vi "EnumeratorUnderstanding.vi"() -> ()   [LabVIEW 2019]
panel:
  out "Value of Enum":enum16{"First ", "Second", "third", ""}(ring)
  in  "Enum":enum16{"First ", "Second", "third", ""}(ring)
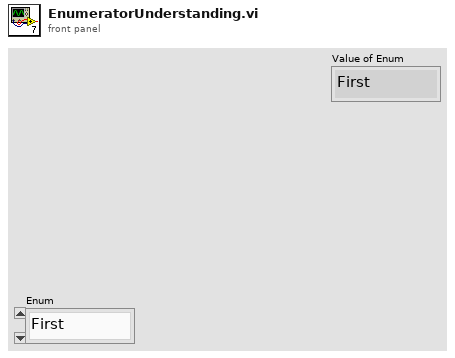
[diagram p1: front panel]
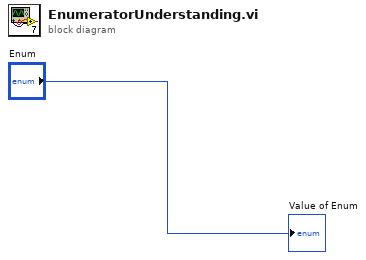
[diagram p0: block diagram]
diagram:
  "Value of Enum" <- "Enum"
